vi "Data Log.vi"(10 "Data In":string[](array[string]), 11 "File Reference In":refnum<file>) -> (3 "File Reference Out":refnum<file>)   [LabVIEW 2016]
doc: "File Path/File Name\nEnter the file path and finally the filename.filetype\n\nData In\nArray of Data to log\n\nColumns\nNumber of Columns to Log\n\nColumn Names\nNames of each column seperated by comma. Need to have same number of names as number of columns."
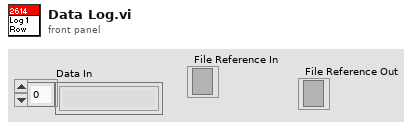
[diagram p1: front panel]
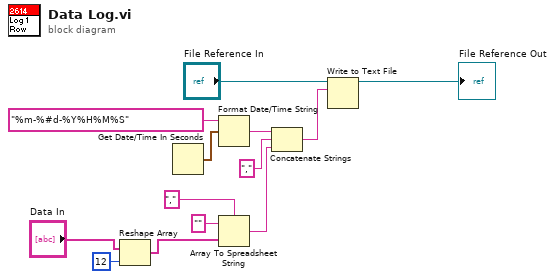
[diagram p0: block diagram]
diagram:
  n1 = Reshape Array("Data In", 12 ("dimension size")) -> (w2:string[])
  n2 = Get Date/Time In Seconds() -> (seconds since 1Jan1904=w9:timestamp)
  n3 = Format Date/Time String(time format string (%c)="%m-%#d-%Y%H%M%S", seconds (now)=w9) -> (date/time string=w7:string)  [unwired: 1 in]
  n4 = Array To Spreadsheet String(delimiter (Tab)=",", array=w2, 3:"" ("format string")) -> (spreadsheet string=w5:string)
  n5 = Concatenate Strings(w7, "," ("string"), w5) -> (w4:string)
  n6 = Write to Text File(file (use dialog)="File Reference In", text=w4) -> (refnum out=→"File Reference Out":refnum<file>)  [unwired: 2 in, 2 out]
